vi "Cosmic Ray Photoshop.vi"(8 "Step Size":dbl=0.037, 11 "Synapse CCD.lvclass In":refnum<class "Synapse CCD.lvclass">) -> (0 "Processed Data":dbl[](array[numeric]), 3 "Synapse CCD.lvclass Out":refnum<class "Synapse CCD.lvclass">)   [LabVIEW 2017, in "Synapse CCD.lvclass"]
uses:
  Synapse CCD.lvclass
  Synapse CCD.lvclass/Synapse CCD.ctl
panel:
  in  "Done Editing":bool
  out "Processed 2":T1(graph)
  in  "Slide":cluster{dbl, dbl}(slide) scale=400.0..600.0
  out "Raw 2":T2(graph)
  in  "Process Full Data Set":bool
  in  "Set Bounds and Process Data":bool
  in  "Upper Bound":dbl=600.0
  in  "Lower Bound":dbl=400.0
  in  "Slope":dbl=9001.0
  out "Processed":T1(graph)
  out "Raw":T2(graph)
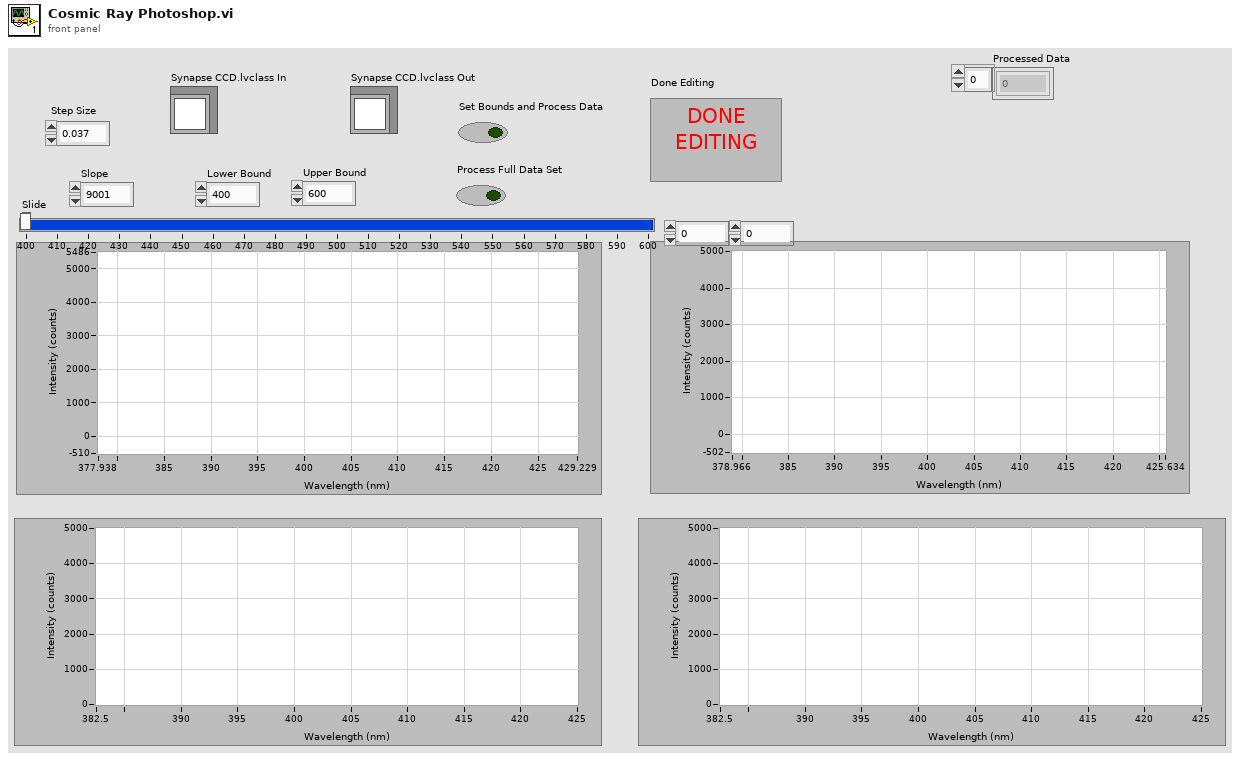
[diagram p1: front panel]
types:
  T1 = cluster{"Array of Wavelengths":dbl[], "Processed Data":dbl[]}
  T2 = cluster{"Array of Wavelengths":dbl[], "Raw Data":i32[]}[]
  T3 = cluster{"Array of Wavelengths":dbl[], "Processed Data":i32[]}
  T4 = cluster{"Array of Wavelengths":dbl[], "Processed Data":i32[]}[]
  T5 = cluster{"Processed Data":dbl[], "Array of Wavelengths":dbl[]}
  T6 = cluster{"Array of Wavelengths":dbl[], "Raw Data":i32[]}
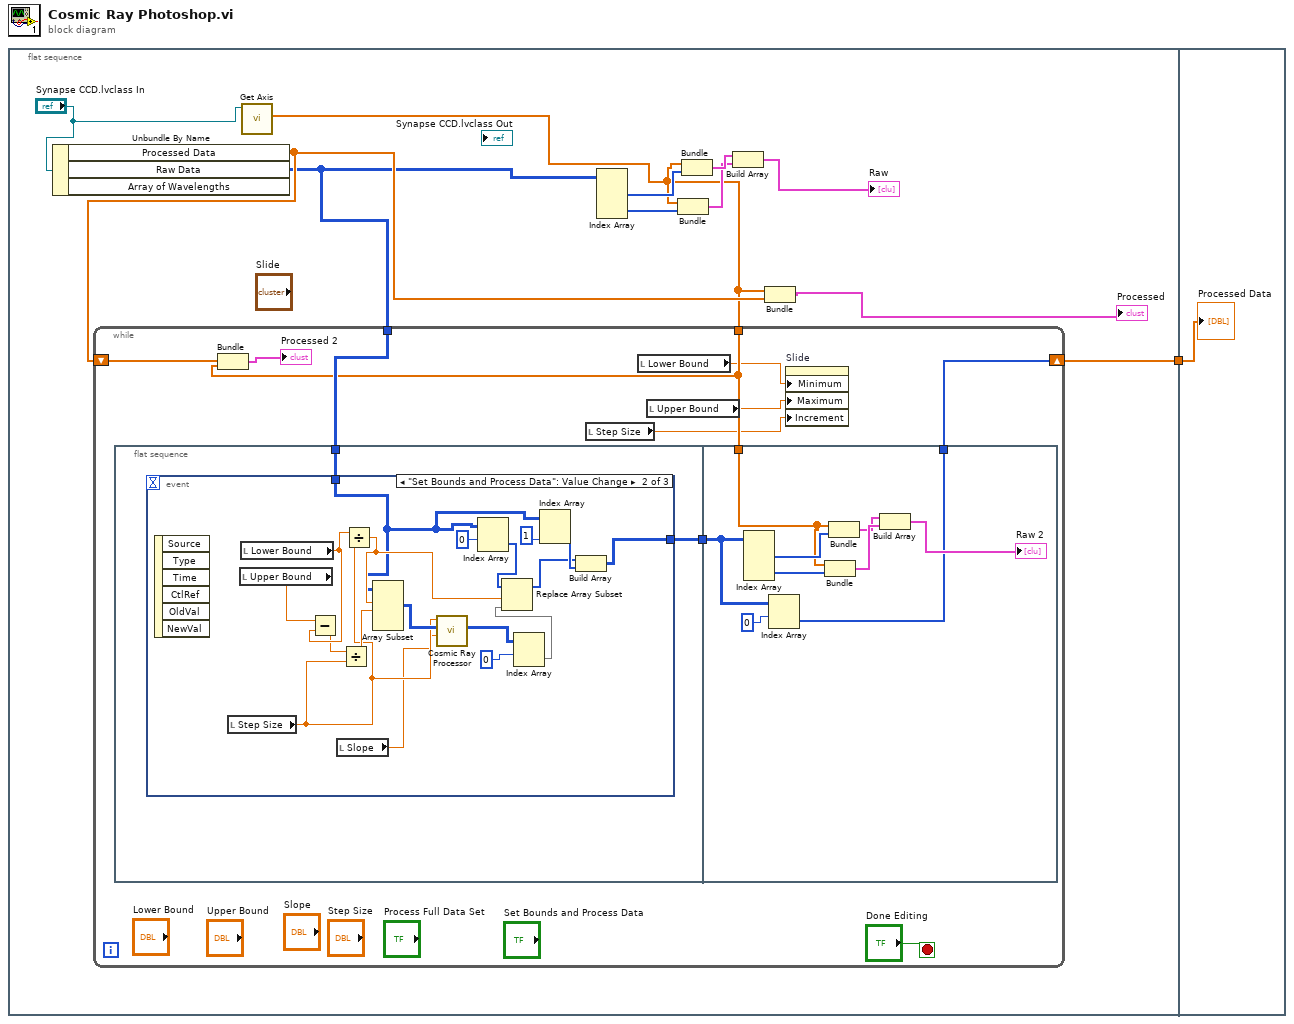
[diagram p0: block diagram]
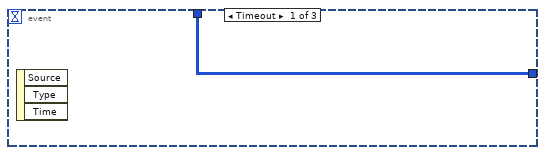
[diagram p2: hidden frame]
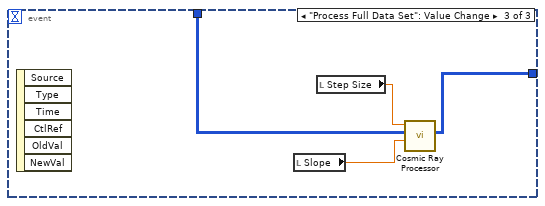
[diagram p3: hidden frame]
diagram:
  n1 = flat-sequence {
    tunnel: [w2] -> w1
    tunnel: w1 -> [w57]
    frame #0 {
      n2 = Unbundle By Name("Synapse CCD.lvclass In") -> ("Processed Data"=w6:dbl[], "Raw Data"=w5:i32[][])  [unwired: 1 out]
      n3 = call "Get Axis.vi"("Synapse CCD.lvclass in"="Synapse CCD.lvclass In") -> ("Array of Wavelengths"=w4:dbl[])  [unwired: 8 in, 2 out]
      n4 = while {
        tunnel: w5 -> [w22]
        shift-right: [w20] -> w2
        shift-left: w6 -> [w19]
        tunnel: w4 -> [w18]
        stop <- "Done Editing" stop-if-true
        n5 = flat-sequence {
          tunnel: w22 -> [w24]
          tunnel: [w23] -> w21
          tunnel: w21 -> [w49]
          tunnel: w18 -> [w51]
          tunnel: [w48] -> w20
          frame #0 {
            n6 = event shown="[1] \"Set Bounds and Process Data\": Value Change" {
              selector: _ -> [_ _ _]
              dyn-events: _ -> [_ _ _]
              timeout: _ -> [_ _ _]
              tunnel: w24 -> [w25 w27 w47]
              tunnel: [w25 w26 w45] -> w23
              event Timeout {
                n7 = event-data() -> ()  [unwired: 1 in, 3 out]
              }
              event "Set Bounds and Process Data": Value Change {
                n8 = event-data() -> ()  [unwired: 1 in, 6 out]
                n9 = local read "Step Size"() -> (w37:dbl)
                n10 = local read "Upper Bound"() -> (w43:dbl)
                n11 = local read "Lower Bound"() -> (w42:dbl)
                n12 = Subtract(x=w43, y=w42) -> (x-y=w41:dbl)
                n13 = local read "Slope"() -> (w36:dbl)
                n14 = Divide(x=w41, y=w37) -> (x/y=w40:dbl)
                n15 = Divide(x=w42, y=w37) -> (x/y=w39:dbl)
                n16 = Array Subset(array=w27, index (row)=w39, length (row)=w40) -> (w38:i32[][])  [unwired: 2 in]
                n17 = call "Cosmic Ray Processor.vi"("Arbitrary Slope Shift"=w36, "Raw Data"=w38, "Step Size"=w37) -> ("Processed Data"=w32:i32[][])  [unwired: 7 in, 1 out]
                n18 = Index Array(array=w27, index (row)=0 ("index")) -> (element=w34:i32[])  [unwired: 1 in]
                n19 = Index Array(array=w32, index (row)=0 ("index")) -> (element=w31:i32[])  [unwired: 1 in]
                n20 = Replace Array Subset(array=w34, new element=w31, index=w39) -> (w28:i32[])
                n21 = Index Array(array=w27, index (col)=1) -> (element=w29:i32[])  [unwired: 1 in]
                n22 = Build Array(w28, w29) -> (w26:i32[][])
              }
              event "Process Full Data Set": Value Change {
                n23 = event-data() -> ()  [unwired: 1 in, 6 out]
                n24 = local read "Slope"() -> (w46:dbl)
                n25 = local read "Step Size"() -> (w44:dbl)
                n26 = call "Cosmic Ray Processor.vi"("Arbitrary Slope Shift"=w46, "Raw Data"=w47, "Step Size"=w44) -> ("Processed Data"=w45:i32[][])  [unwired: 7 in, 1 out]
              }
            }
          }
          frame #1 {
            n27 = Index Array(array=w49) -> (element #1=w52:i32[], element #2=w54:i32[])  [unwired: 4 in]
            n28 = Index Array(array=w49, index (row)=0 ("index")) -> (element=w48:i32[])  [unwired: 1 in]
            n29 = Bundle("Array of Wavelengths"=w51, "Processed Data"=w54) -> (w55:T3)  [unwired: 1 in]
            n30 = Bundle("Array of Wavelengths"=w51, "Processed Data"=w52) -> (w53:T3)  [unwired: 1 in]
            n31 = Build Array(w53, w55) -> (→"Raw 2":T4)
          }
        }
        n32 = Bundle("Processed Data"=w19, "Array of Wavelengths"=w18) -> (→"Processed 2":T5)  [unwired: 1 in]
        n33 = local read "Step Size"() -> (w13:dbl)
        n34 = local read "Lower Bound"() -> (w14:dbl)
        n35 = local read "Upper Bound"() -> (w15:dbl)
        n36 = property on="Slide" class="Slide (strict)"("Minimum"=w14, "Maximum"=w15, "Increment"=w13) -> ()  [unwired: 2 in, 2 out]
      }
      n37 = Index Array(array=w5) -> (element #1=w11:i32[], element #2=w9:i32[])  [unwired: 4 in]
      n38 = Bundle("Array of Wavelengths"=w4, "Raw Data"=w9) -> (w8:T6)  [unwired: 1 in]
      n39 = Bundle("Array of Wavelengths"=w4, "Raw Data"=w11) -> (w10:T6)  [unwired: 1 in]
      n40 = Build Array(w10, w8) -> (→"Raw":T2)
      n41 = Bundle("Array of Wavelengths"=w4, "Processed Data"=w6) -> (→"Processed":T1)  [unwired: 1 in]
    }
    frame #1 {
      "Processed Data" <- w57
    }
  }
